vi "List Definitions.vi"(7 "Type":string, 8 "error in (no error)":errorcluster, 9 "Listbox Refnum":refnum<vi>, 11 "InsightCM Console Wrapper in":refnum<class "InsightCM Console Wrapper.lvclass">) -> (0 "error out":errorcluster, 3 "InsightCM Console Wrapper out":refnum<class "InsightCM Console Wrapper.lvclass">)   [LabVIEW 2020, in "InsightCM Console Wrapper.lvclass"]
doc: "This VI returns a list of definitions in the server based on a type entry.\n\nConsole command -> listdefinitions -t [type]"
uses:
  InsightCM Console Wrapper.lvclass
  C:/Users/fflores/Documents/GitHub Projects/LabVIEW-CLI-Wrapper/Console Wrapper/Console Wrapper.lvclass
  Console Wrapper/Console Wrapper.lvclass/Console Wrapper.ctl
  Console Wrapper/Write Command Options.vi
  Console Wrapper/Write Command.vi
  Console Wrapper/Console Wrapper.lvclass
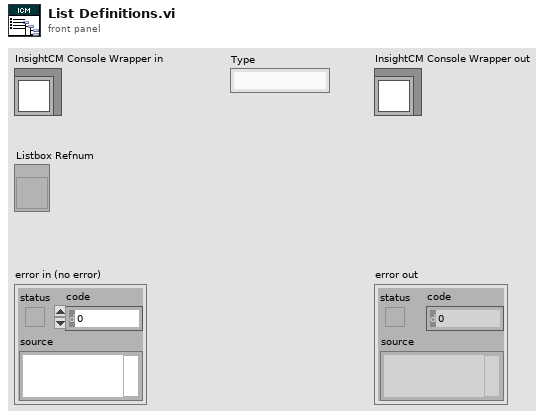
[diagram p1: front panel]
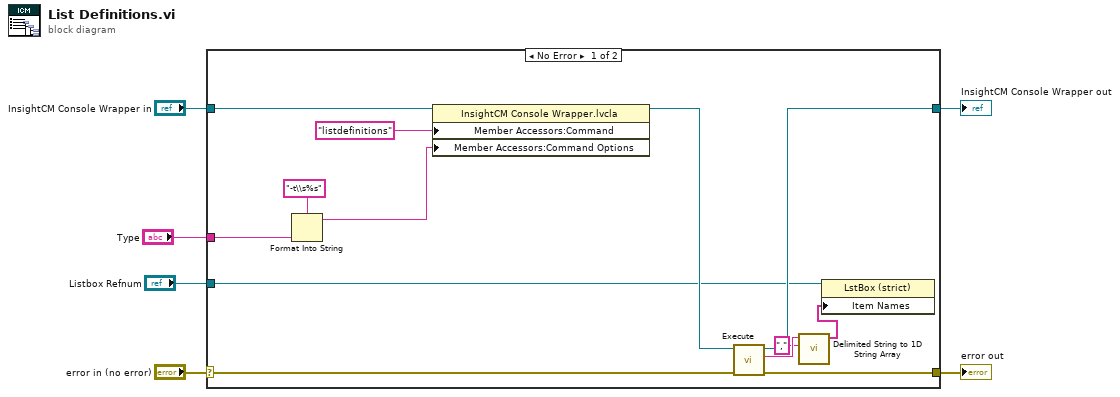
[diagram p0: block diagram]
diagram:
  n1 = case shown="No Error" "error in (no error)" {
    selector: "error in (no error)" -> [w18 w21]
    tunnel: [w17 w21] -> w5
    tunnel: [w15 w20] -> w3
    tunnel: "InsightCM Console Wrapper in" -> [w19 w20]
    tunnel: "Type" -> [w9 _]
    tunnel: "Listbox Refnum" -> [w13 _]
    frame No Error {
      n2 = Format Into String(format string="-t\\s%s", w9) -> (resulting string=w7:string)  [unwired: 2 in, 1 out]
      n3 = property class="InsightCM Console Wrapper.lvcla"(reference=w19, "Member Accessors:Command"="listdefinitions" ("Command"), "Member Accessors:Command Options"=w7) -> (reference out=w16:refnum<class "InsightCM Console Wrapper.lvclass">)  [unwired: 1 in, 1 out]
      n4 = call "Execute.vi"("error in (no error)"=w18, "Console Wrapper in"=w16) -> ("error out"=w17:errorcluster, "Command output"=w11:string, "Console Wrapper out"=w15:refnum<class "InsightCM Console Wrapper.lvclass">)  [unwired: 7 in]
      n5 = call <vilib>:"Delimited String to 1D String Array.vi"("delimiter"=",", "delimited string"=w11) -> ("string array"=w12:string[])  [unwired: 9 in]
      n6 = property class="LstBox (strict)"(reference=w13, "Item Names"=w12) -> ()  [unwired: 1 in, 2 out]
    }
    frame Error {
    }
  }
  "error out" <- w5
  "InsightCM Console Wrapper out" <- w3
